vi "案例.vi"() -> ()   [LabVIEW 2018]
panel:
  out "数组 2":string[](array[string])
  in  "数组":string[](array[string])
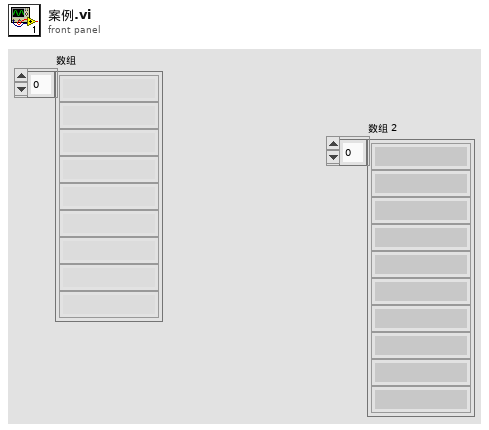
[diagram p1: front panel]
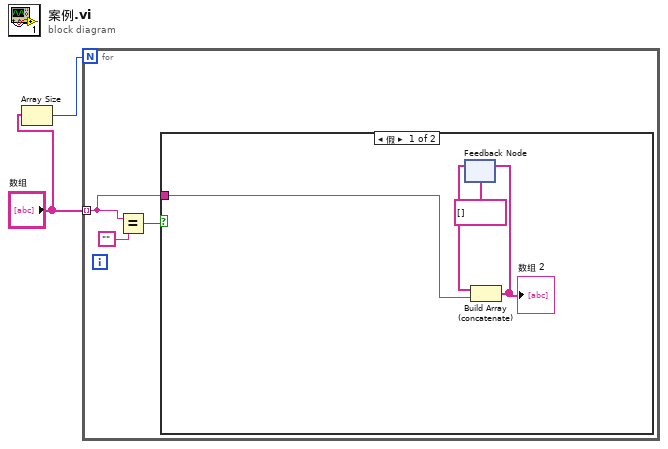
[diagram p0: block diagram]
diagram:
  n1 = Array Size(array="数组") -> (size(s)=w2:i32)
  n2 = for {
    N: w2 -> [_]
    tunnel: "数组" -> [w3] mode=indexing
    n3 = Equal?(x=w3, y="") -> (x = y?=w4:bool)
    n4 = case shown="假" w4 {
      tunnel: w3 -> [w9 _]
      frame False {
        n5 = feedback #1(string[] []) -> (w8:string[])
        n6 = Build Array (concatenate)(w8, w9) -> (w7:string[])
        "数组 2" <- w7
        n7 = feedback-in #1(w7) -> ()
      }
      frame True {
      }
    }
  }
